vi "Series from multiple channels.vi"(8 "Row Numbers":i32[](array[numeric]), 9 "Ordinate Index":i32, 11 "Channel Values":string[][](array[string])) -> (0 "Plot?":bool, 1 "Row Numbers Out":i32[](array[numeric]), 2 "Averaged Values":dbl[](array[numeric]), 3 "Positions":dbl[](array[numeric]))   [LabVIEW 2015]
uses:
  <vilib>/Analysis/baseanly.llb/Mean (DBL).vi
  Results_plotter_Global.vi
  <vilib>/Analysis/NI_AALBase.lvlib
panel:
  out "No of table rows":i32
  out "Number of plot values":i32
  out "Channels":string[](array[string])
  out "element":string
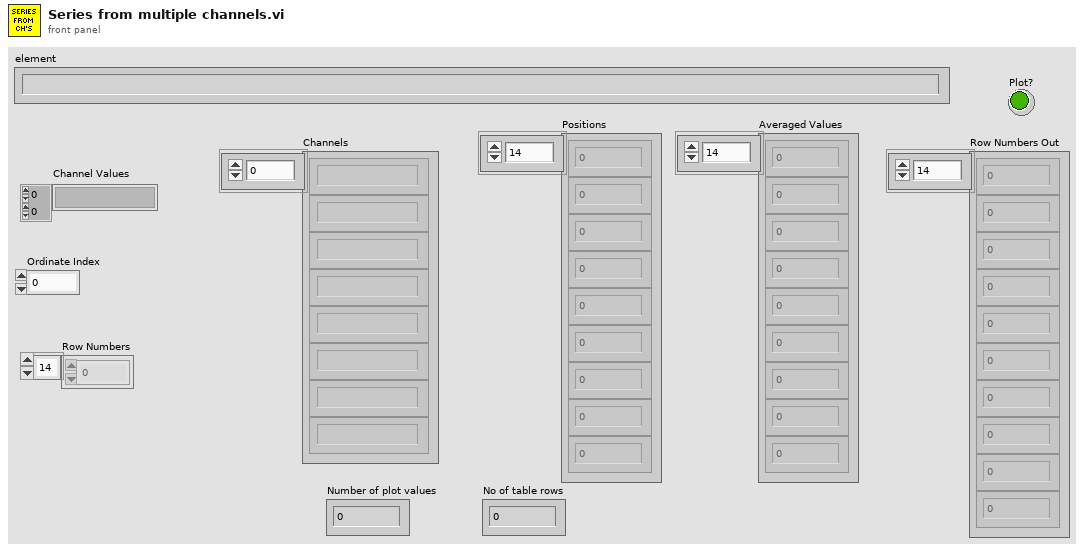
[diagram p1: front panel]
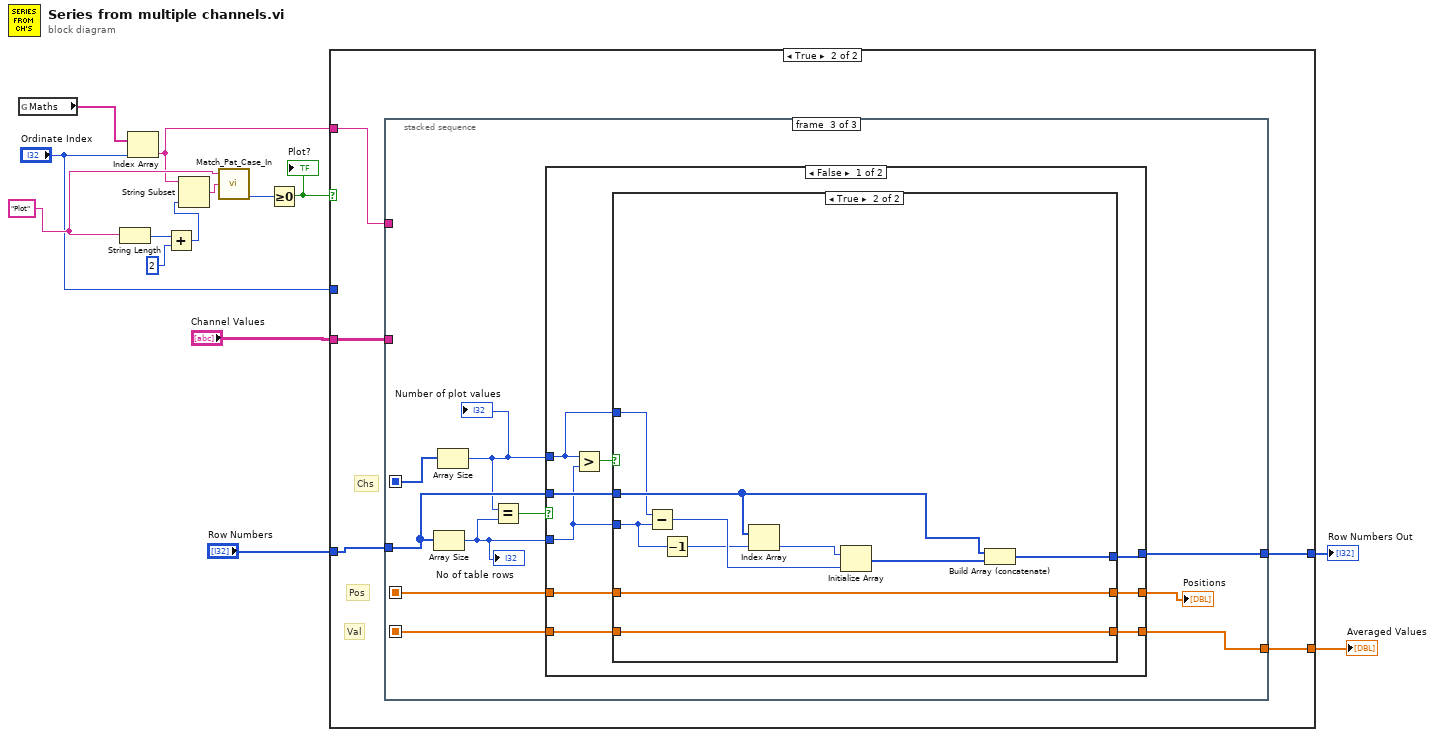
[diagram p0: block diagram]
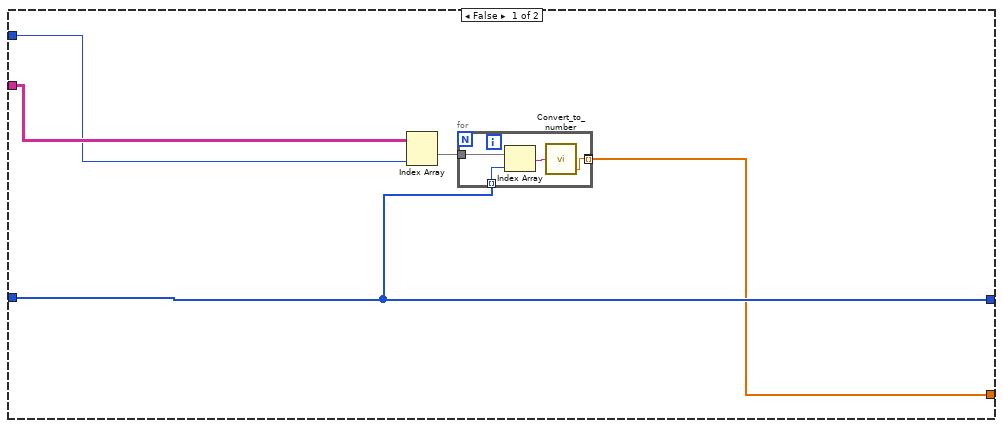
[diagram p2: hidden frame]
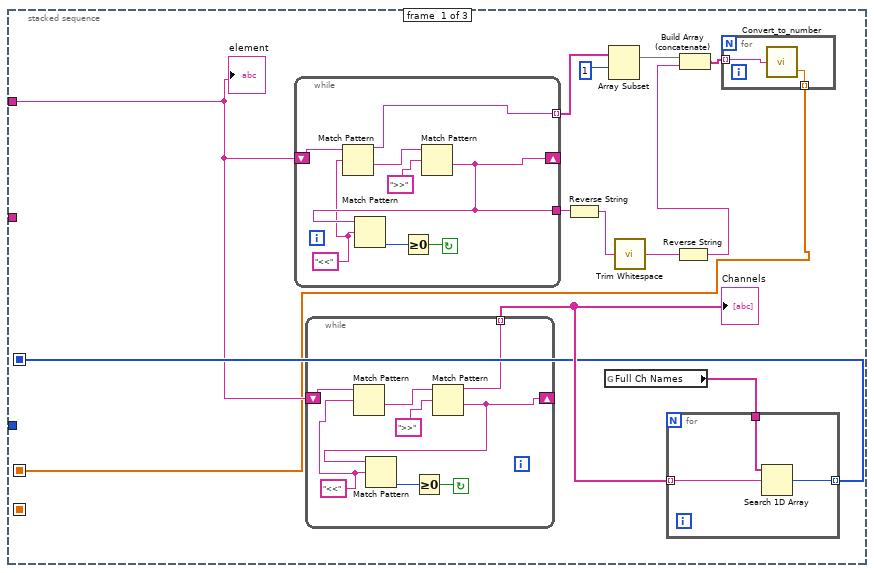
[diagram p3: hidden frame]
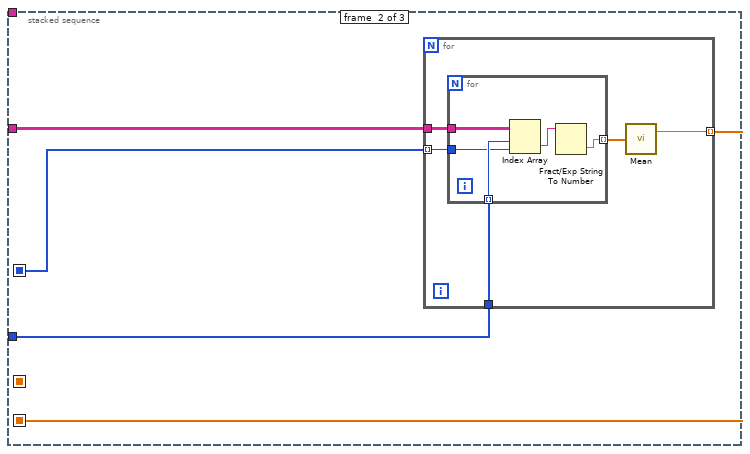
[diagram p4: hidden frame]
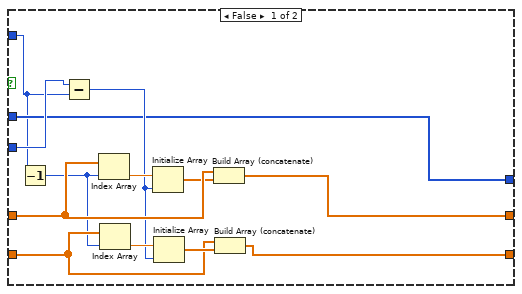
[diagram p5: hidden frame]
diagram:
  w8 = "Plot" ("regular expression")
  n1 = global read "Results_plotter_Global.vi" "Maths"() -> (w9:string[])
  n2 = String Length(string=w8) -> (length=w11:i32)
  n3 = Index Array(array=w9, index="Ordinate Index") -> (element=w6:string)
  n4 = Add(x=w11, y=2) -> (x+y=w13:i32)
  n5 = String Subset(string=w6, length (rest)=w13) -> (substring=w14:string)  [unwired: 1 in]
  n6 = call "Match_Pat_Case_In.vi"("String to match"=w8, "String"=w14) -> ("offset past match"=w10:i32)  [unwired: 1 in, 3 out]
  n7 = Greater Or Equal To 0?(x=w10) -> (x >= 0?=w7:bool)
  "Plot?" <- w7
  n8 = case shown="True" w7 {
    tunnel: "Channel Values" -> [w18 w28]
    tunnel: w6 -> [_ w27]
    tunnel: "Row Numbers" -> [w17 w26]
    tunnel: [w17 w25] -> w4
    tunnel: [w16 w24] -> w2
    tunnel: "Ordinate Index" -> [w15 _]
    frame False {
      n9 = Index Array(array=w18, index (col)=w15) -> (element=w19:string[])  [unwired: 1 in]
      n10 = for {
        tunnel: w17 -> [w23] mode=indexing
        tunnel: w19 -> [w22]
        tunnel: [w20] -> w16 mode=indexing
        tunnel: [w20] -> _ mode=indexing
        n11 = Index Array(array=w22, index=w23) -> (element=w21:string)
        n12 = call "Convert_to_number.vi"("string"=w21) -> ("Number"=w20:dbl)  [unwired: 1 out]
      }
    }
    frame True {
      # "Val"
      # "Pos"
      # "Chs"
      n13 = stacked-sequence {
        seq-local: [w32 _ _] -> [_ w65 w86]
        seq-local: [w29 _ _] -> [_ _ w82]
        seq-local: [_ w63 _] -> [_ _ w81]
        tunnel: w28 -> [_ w66 _]
        tunnel: w27 -> [w31 _ _]
        tunnel: w26 -> [_ w64 w83]
        tunnel: [_ _ w84] -> w25
        tunnel: [_ _ w78] -> w24
        frame #0 {
          n14 = while {
            shift-left: w31 -> [w62]
            shift-right: [w57] -> _
            tunnel: [w58] -> w35 mode=indexing
            tunnel: [w57] -> w38
            stop <- w59 continue-if-true
            w56 = "<<" ("regular expression")
            n15 = Match Pattern(string=w62, regular expression=w56) -> (before substring=w58:string, after substring=w61:string)  [unwired: 3 out]
            n16 = Match Pattern(string=w61, regular expression=">>") -> (after substring=w57:string)  [unwired: 4 out]
            n17 = Match Pattern(string=w57, regular expression=w56) -> (offset past match=w60:i32)  [unwired: 4 out]
            n18 = Greater Or Equal To 0?(x=w60) -> (x >= 0?=w59:bool)
          }
          n19 = while {
            tunnel: [w49] -> w33 mode=indexing
            shift-left: w31 -> [w54]
            shift-right: [w52] -> _
            stop <- w50 continue-if-true
            w48 = "<<" ("regular expression")
            n20 = Match Pattern(string=w54, regular expression=w48) -> (after substring=w53:string)  [unwired: 4 out]
            n21 = Match Pattern(string=w53, regular expression=">>") -> (before substring=w49:string, after substring=w52:string)  [unwired: 3 out]
            n22 = Match Pattern(string=w52, regular expression=w48) -> (offset past match=w51:i32)  [unwired: 4 out]
            n23 = Greater Or Equal To 0?(x=w51) -> (x >= 0?=w50:bool)
          }
          "Channels" <- w33
          n24 = Reverse String(1:w38) -> (0:w39:string)
          n25 = global read "Results_plotter_Global.vi" "Full Ch Names"() -> (w34:string[])
          n26 = Array Subset(array=w35, index=1) -> (w36:string[])  [unwired: 1 in]
          n27 = call <vilib>:"Trim Whitespace.vi"("string"=w39) -> ("trimmed string"=w40:string)  [unwired: 1 in]
          n28 = for {
            tunnel: w34 -> [w46]
            tunnel: w33 -> [w45] mode=indexing
            tunnel: [w44] -> w32 mode=indexing
            n29 = Search 1D Array(1D array=w46, element=w45) -> (index of element=w44:i32)  [unwired: 1 in]
          }
          n30 = Reverse String(1:w40) -> (0:w41:string)
          n31 = Build Array (concatenate)(w36, w41) -> (w30:string[])
          n32 = for {
            tunnel: w30 -> [w43] mode=indexing
            tunnel: [w42] -> w29 mode=indexing
            n33 = call "Convert_to_number.vi"("string"=w43) -> ("Number"=w42:dbl)  [unwired: 1 out]
          }
          "element" <- w31
        }
        frame #1 {
          n34 = for {
            tunnel: w66 -> [w71]
            tunnel: w64 -> [w70]
            tunnel: w65 -> [w69] mode=indexing
            tunnel: [w67] -> w63 mode=indexing
            n35 = for {
              tunnel: w71 -> [w76]
              tunnel: w70 -> [w75] mode=indexing
              tunnel: w69 -> [w74]
              tunnel: [w72] -> w68 mode=indexing
              n36 = Index Array(array=w76, index (row)=w75, index (col)=w74) -> (element=w73:string)
              n37 = Fract/Exp String To Number(string=w73) -> (number=w72:dbl)  [unwired: 3 in, 1 out]
            }
            n38 = call-poly <vilib>:"Mean.vi"("X"=w68) -> ("mean"=w67:dbl)  [unwired: 1 out]
          }
        }
        frame #2 {
          n39 = Array Size(array=w83) -> (size(s)=w79:i32)
          "No of table rows" <- w79
          n40 = Array Size(array=w86) -> (size(s)=w80:i32)
          "Number of plot values" <- w80
          n41 = Equal?(x=w80, y=w79) -> (x = y?=w85:bool)
          n42 = case shown="False" w85 {
            tunnel: [w89 w121] -> w84
            tunnel: w83 -> [w90 w121]
            tunnel: [w94 w120] -> w77
            tunnel: w82 -> [w93 w120]
            tunnel: [w92 w119] -> w78
            tunnel: w81 -> [w91 w119]
            tunnel: w80 -> [w88 _]
            tunnel: w79 -> [w87 _]
            frame False {
              n43 = Greater?(x=w88, y=w87) -> (0:w95:bool)
              n44 = case shown="True" w95 {
                tunnel: [w106 w118] -> w94
                tunnel: w93 -> [w107 w118]
                tunnel: [w99 w117] -> w92
                tunnel: w91 -> [w100 w117]
                tunnel: w90 -> [w98 w115]
                tunnel: [w98 w116] -> w89
                tunnel: w88 -> [w97 w114]
                tunnel: w87 -> [w108 w111]
                frame False {
                  n45 = Decrement(x=w97) -> (x-1=w96:i32)
                  n46 = Subtract(x=w108, y=w97) -> (x-y=w101:i32)
                  n47 = Index Array(array=w107, index=w96) -> (element=w104:dbl)
                  n48 = Index Array(array=w100, index=w96) -> (element=w103:dbl)
                  n49 = Initialize Array(w104, w101) -> (w105:dbl[])
                  n50 = Initialize Array(w103, w101) -> (w102:dbl[])
                  n51 = Build Array (concatenate)(w107, w105) -> (w106:dbl[])
                  n52 = Build Array (concatenate)(w100, w102) -> (w99:dbl[])
                }
                frame True {
                  n53 = Subtract(x=w114, y=w111) -> (x-y=w110:i32)
                  n54 = Decrement(x=w111) -> (x-1=w109:i32)
                  n55 = Index Array(array=w115, index=w109) -> (element=w113:i32)
                  n56 = Initialize Array(w113, w110) -> (w112:i32[])
                  n57 = Build Array (concatenate)(w115, w112) -> (w116:i32[])
                }
              }
            }
            frame True {
            }
          }
          "Positions" <- w77
        }
      }
    }
  }
  "Row Numbers Out" <- w4
  "Averaged Values" <- w2
